vi "get_motor_info.vi"(8 "error in (no error)":errorcluster caption="错误输入（无错误）", 11 "StepMotor 输入":refnum<class "StepMotor.lvclass">) -> (0 "error out":errorcluster caption="错误输出", 2 "motion":T1, 3 "StepMotor 输出":refnum<class "StepMotor.lvclass">)   [LabVIEW 2016, in "MotionControl.lvlib" / "StepMotor.lvclass"]
uses:
  <userlib>/MotionControl/StepMotor/StepMotor.lvclass
  <userlib>/MotionControl/StepMotor/StepMotor.lvclass/StepMotor.ctl
  <userlib>/UISimCanFunc_wrapper/UISimCanFunc_wrapper.lvlib
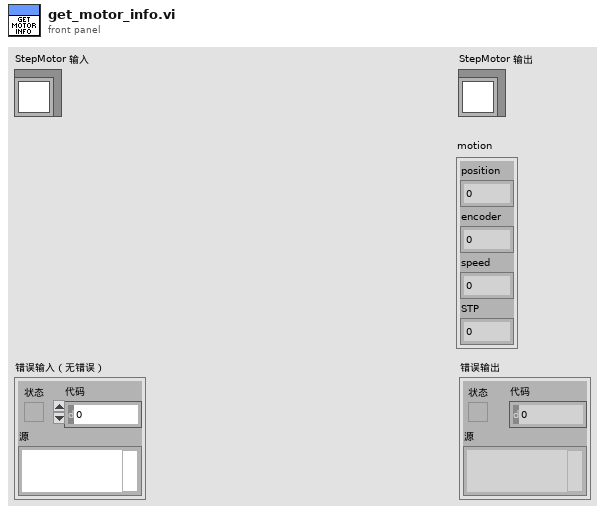
[diagram p1: front panel]
types:
  T1 = cluster{"position":i32, "encoder":i32, "speed":i32, "STP":i32}
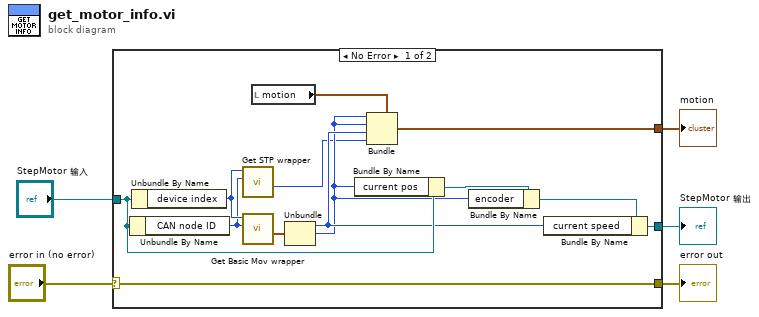
[diagram p0: block diagram]
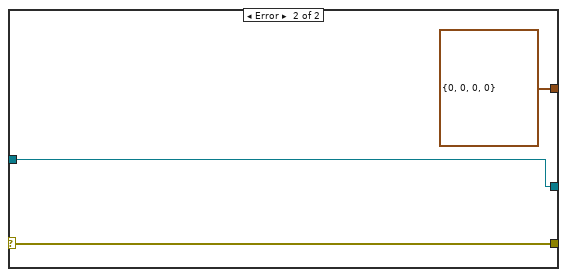
[diagram p2: hidden frame]
diagram:
  n1 = case shown="No Error" "error in (no error)" {
    selector: "error in (no error)" -> [w18 w21]
    tunnel: [w18 w21] -> w4
    tunnel: [w14 w20] -> w2
    tunnel: "StepMotor 输入" -> [w17 w20]
    tunnel: [w12 cluster{i32, i32, i32, i32} {0, 0, 0, 0}] -> w1
    frame No Error {
      n2 = Unbundle By Name(w17) -> ("CAN node ID"=w7:u32)
      n3 = Unbundle By Name(w17) -> ("device index"=w8:u32)
      n4 = call <userlib>:"Get STP wrapper.vi"("dwCanNodeId"=w7, "dwDevIndex"=w8) -> ("pRtnValue out"=w6:i32)  [unwired: 7 in, 2 out]
      n5 = call <userlib>:"Get Basic Mov wrapper.vi"("dwCanNodeId"=w7, "dwDevIndex"=w8) -> ("pBasicMovObj out"=w13:cluster{"iSpd":i32, "iPos":i32, "iTimeOut":i32})  [unwired: 7 in, 2 out]
      n6 = local read "motion"() -> (w11:T1)
      n7 = Unbundle(w13) -> ("iSpd"=w10:i32, "iPos"=w9:i32)  [unwired: 1 out]
      n8 = Bundle By Name(cluster=w17, "current pos"=w9) -> (w16:refnum<class "StepMotor.lvclass">)
      n9 = Bundle(cluster=w11, "position"=w9, "encoder"=w9, "speed"=w10, "STP"=w6) -> (w12:T1)
      n10 = Bundle By Name(cluster=w16, "encoder"=w9) -> (w15:refnum<class "StepMotor.lvclass">)
      n11 = Bundle By Name(cluster=w15, "current speed"=w10) -> (w14:refnum<class "StepMotor.lvclass">)
    }
    frame Error {
    }
  }
  "error out" <- w4
  "StepMotor 输出" <- w2
  "motion" <- w1
